vi "toStop.vi"(0 "Left":i16, 5 "Distance to street":dbl, 7 "Booleanos e Contadores Iniciais IN":T1={"Correct"=FALSE, "Enable State change"=TRUE, "First End"=FALSE, "Intersections crossed"=0.0, "Intersections crossed total"=0.0} caption="Booleanos e Contadores", 9 "Características in":T3={"Colors and Directions"=[enum."Zero", enum."Zero", enum."Zero", enum."Zero", enum."Zero", enum."Zero"], "Direction"=enum."Right", "CS"=enum."Street", "Old Color"=enum."White"}, 11 "Right":i16) -> (3 "Boolean":bool, 8 "Booleanos e Contadores Iniciais OUT":T1={"Correct"=FALSE, "Enable State change"=TRUE, "First End"=FALSE, "Intersections crossed"=0.0, "Intersections crossed total"=0.0} caption="Booleanos e Contadores", 10 "Características out":T3={"Colors and Directions"=[enum."Zero", enum."Zero", enum."Zero", enum."Zero", enum."Zero", enum."Zero"], "Direction"=enum."Right", "CS"=enum."Street", "Old Color"=enum."White"}, 12 "Enable 2":bool)   [LabVIEW 2016]
uses:
  <vilib>/NXT/Subs/ColorSensorColors.ctl
  booleanos.ctl
panel:
  # "Permite que ocorra troca \nde estados se True e interrompe-as \nse False."
  # "Booleano que retorna F quando chega em Delivery.\nGarantindo que não contará\nmais intersections"
  # "Salva o total de interseções \ncruzadas"
  # "Contador de quantas \ninterseções foram cruzadas.\nSoma ao acertar"
  # "Permite que ocorra troca \nde estados se True e interrompe-as \nse False."
  # "Booleano que retorna F quando chega em Delivery.\nGarantindo que não contará\nmais intersections"
  # "Salva o total de interseções \ncruzadas"
  # "Contador de quantas \ninterseções foram cruzadas.\nSoma ao acertar"
  # "black"
  # "blue"
  # "green"
  # "yellow"
  # "red"
  # "black"
  # "blue"
  # "green"
  # "yellow"
  # "red"
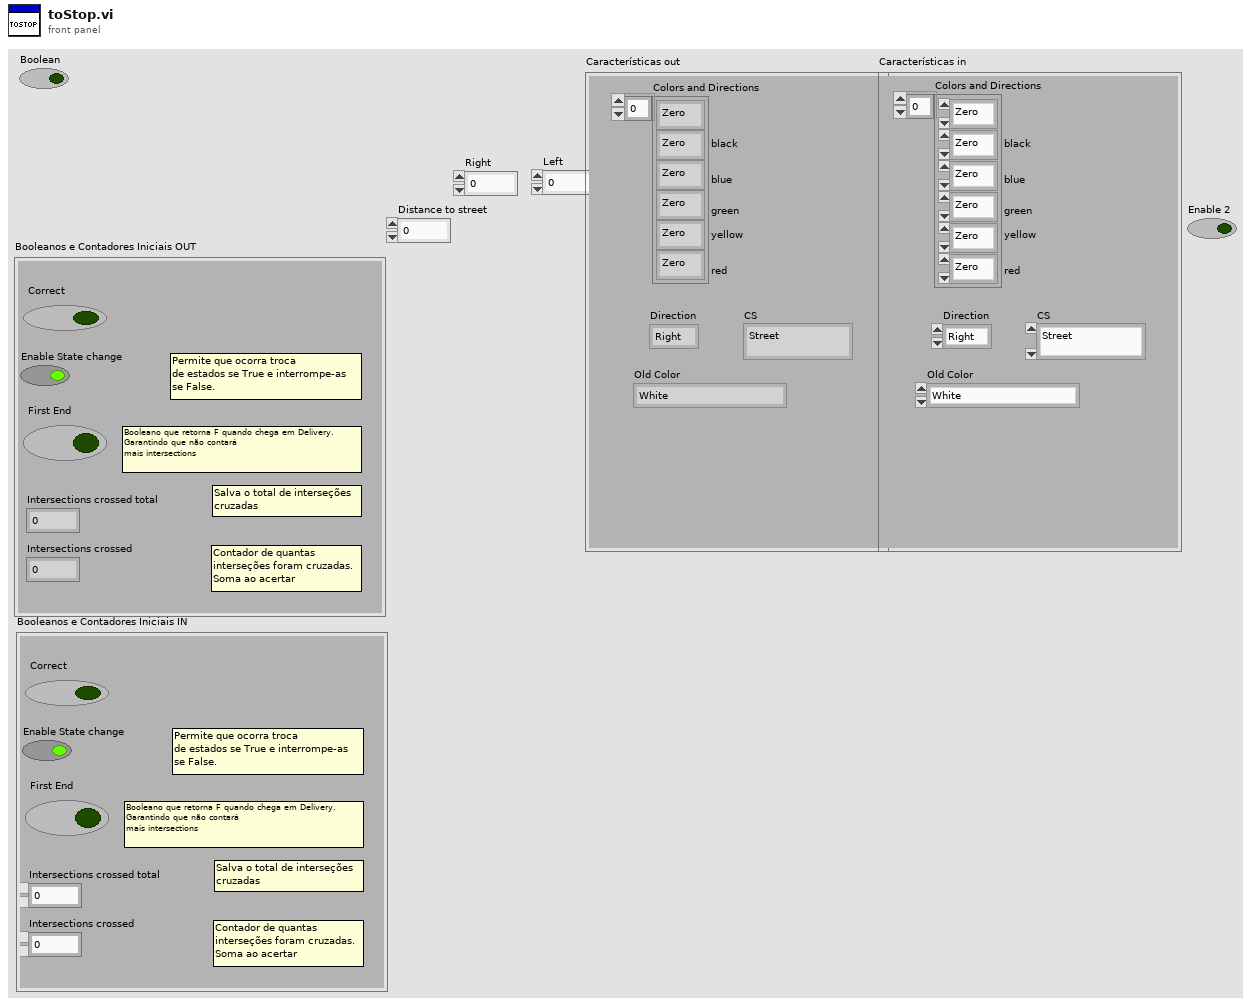
[diagram p1: front panel]
types:
  T1 = typedef "booleanos.ctl" = cluster{"Correct":bool, "Enable State change":bool, "First End":bool, "Intersections crossed":dbl, "Intersections crossed total":dbl}
  T2 = typedef "ColorSensorColors.ctl" = enum16{"No Color", "Black", "Blue", "Green", "Yellow", "Red", "White", "Brown"}
  T3 = cluster{"Colors and Directions":enum16{"Zero", "Right", "Front", "Left"}[], "Direction":enum16{"Zero", "Right", "Front", "Left"}, "CS":enum16{"Street", "Intersection", "End", "Stop", "Square", "Delivery"}, "Old Color":T2}
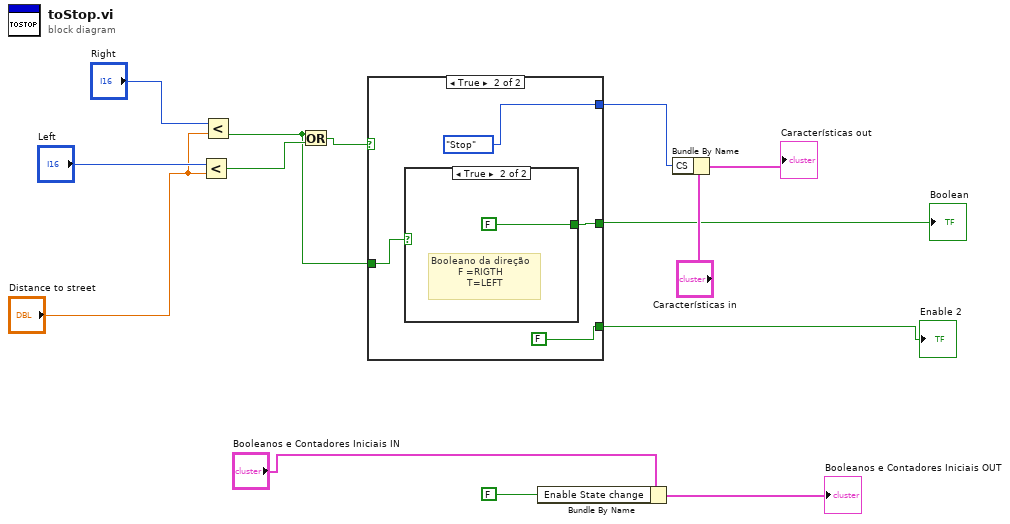
[diagram p0: block diagram]
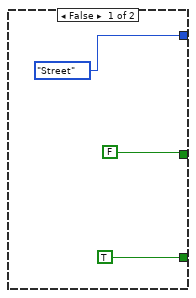
[diagram p2: hidden frame]
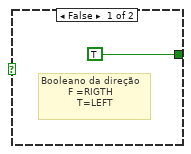
[diagram p3: hidden frame]
diagram:
  n1 = Less?(x="Left", y="Distance to street") -> (x < y?=w14:bool)
  n2 = Less?(x="Right", y="Distance to street") -> (x < y?=w7:bool)
  n3 = Or(x=w7, y=w14) -> (x .or. y?=w13:bool)
  n4 = case shown="True" w13 {
    tunnel: [enum16{"Street", "Intersection", "End", "Stop"}."Street" ("CS") enum16{"Street", "Intersection", "End", "Stop"}."Stop" ("CS")] -> w8
    tunnel: w7 -> [_ w20]
    tunnel: [FALSE w19] -> w6
    tunnel: [TRUE FALSE] -> w1
    frame False {
    }
    frame True {
      n5 = case shown="True" w20 {
        tunnel: [TRUE FALSE] -> w19
        frame False {
          # "Booleano da direção\n         F =RIGTH\n            T=LEFT"
        }
        frame True {
          # "Booleano da direção\n         F =RIGTH\n            T=LEFT"
        }
      }
    }
  }
  "Boolean" <- w6
  "Enable 2" <- w1
  n6 = Bundle By Name(cluster="Booleanos e Contadores Iniciais IN", "Enable State change"=FALSE) -> (→"Booleanos e Contadores Iniciais OUT":T1)
  n7 = Bundle By Name(cluster="Características in", "CS"=w8) -> (→"Características out":T3)
